vi "CallPython.vi"() -> ()   [LabVIEW 2013]
panel:
  out "standard output":string caption="Standardausgabe"
  out "return code":i32 caption="Fehlercode"
  out "error out":errorcluster caption="Fehler (Ausgang)"
  in  "error in (no error)":errorcluster caption="Fehler (Eingang, kein Fehler)"
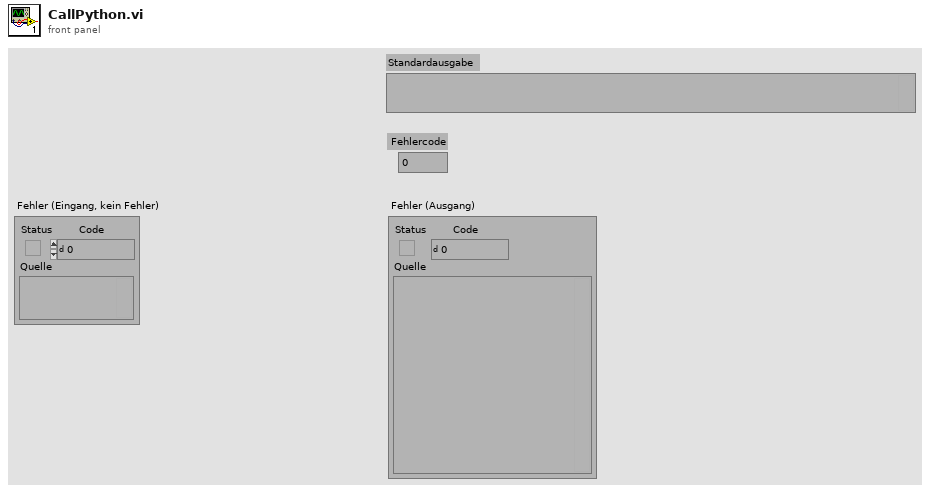
[diagram p1: front panel]
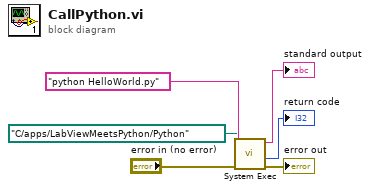
[diagram p0: block diagram]
diagram:
  n1 = call <vilib>:"System Exec.vi"("error in (no error)"="error in (no error)", "working directory"=path "C:/apps/LabViewMeetsPython/Python", "command line"="python HelloWorld.py") -> ("error out"=→"error out":errorcluster, "return code"=→"return code":i32, "standard output"=→"standard output":string)  [unwired: 5 in, 1 out]
